vi "Draw.vi"(8 "error in (no error)":errorcluster, 11 "reference in":refnum<class "Pgui_Obj.lvclass">) -> (0 "error out":errorcluster, 2 "Draw Instr":picture, 3 "reference out":refnum<class "Pgui_Obj.lvclass">)   [LabVIEW 2019, in "Pgui_Obj.lvclass"]
uses:
  Pgui_Obj.lvclass
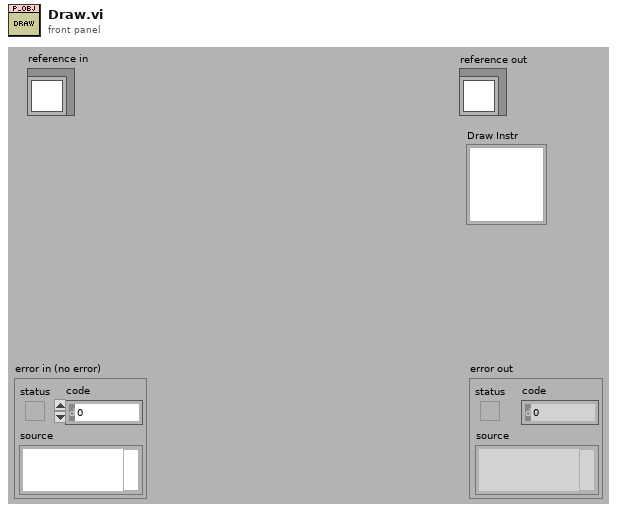
[diagram p1: front panel]
types:
  T1 = typedef "Pgui_Obj.lvclass/ObjectAttributes.ctl" = cluster{"Children":refnum<class "Pgui_Obj.lvclass">[], "Draw Instr":picture, "Params":cluster{"left":i16, "top":i16, "right":i16, "bottom":i16}, "Parent_Pgui_Obj":refnum<class "Pgui_Obj.lvclass">, "MouseOver":bool}
  T2 = cluster{"left":i16, "top":i16, "right":i16, "bottom":i16}
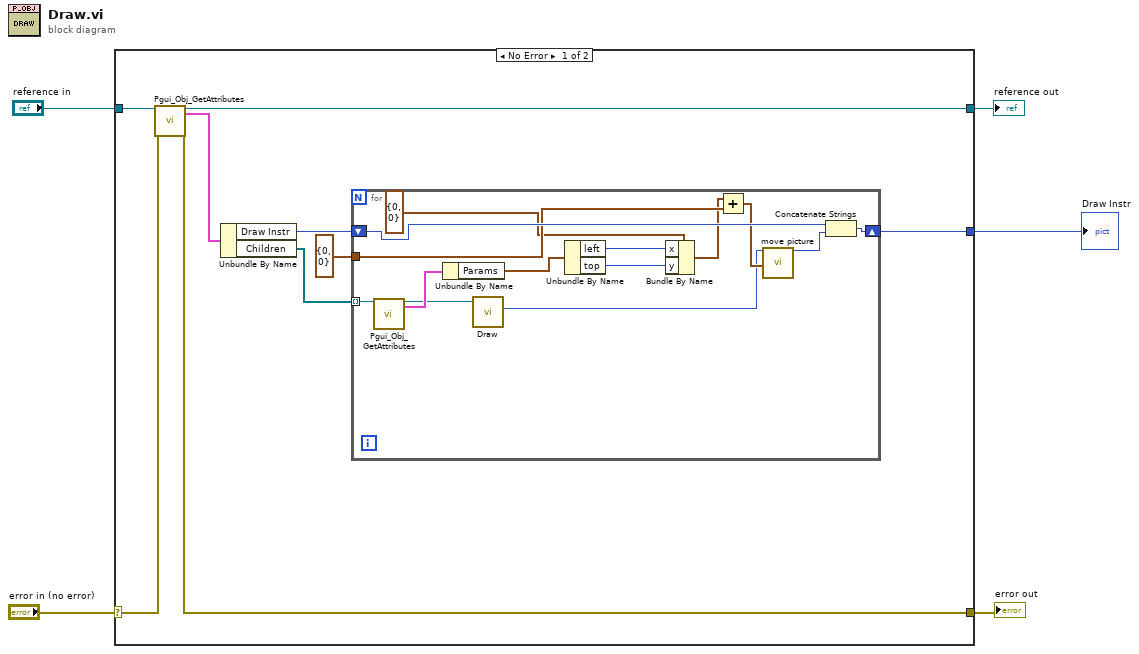
[diagram p0: block diagram]
diagram:
  n1 = case shown="No Error" "error in (no error)" {
    selector: "error in (no error)" -> [w14 w30]
    tunnel: [w12 w30] -> w4
    tunnel: [w10 w29] -> w2
    tunnel: "reference in" -> [w11 w29]
    tunnel: [w6 _] -> w1
    frame No Error {
      n2 = call "Pgui_Obj_GetAttributes.vi"("reference in"=w11, "error in (no error)"=w14) -> ("reference out"=w10:refnum<class "Pgui_Obj.lvclass">, "Data"=w13:T1, "error out"=w12:errorcluster)  [unwired: 14 in, 1 out]
      n3 = Unbundle By Name(w13) -> ("Draw Instr"=w9:picture, "Children"=w7:refnum<class "Pgui_Obj.lvclass">[])
      n4 = for {
        tunnel: w7 -> [w18] mode=indexing
        shift-right: [w28] -> w6
        shift-left: w9 -> [w26]
        tunnel: cluster{"x":i16, "y":i16} {"x"=0, "y"=0} ("input cluster") -> [w22]
        n5 = call "Pgui_Obj_GetAttributes.vi"("reference in"=w18) -> ("reference out"=w16:refnum<class "Pgui_Obj.lvclass">, "Data"=w17:T1)  [unwired: 15 in, 2 out]
        n6 = Unbundle By Name(w17) -> ("Params"=w25:T2)
        n7 = call-dynamic "Draw.vi"("reference in"=w16) -> ("Draw Instr"=w15:picture)  [unwired: 8 in, 2 out]
        n8 = Unbundle By Name(w25) -> ("left"=w24:i16, "top"=w23:i16)
        n9 = Bundle By Name(cluster=cluster{"x":i16, "y":i16} {"x"=0, "y"=0} ("move"), "x"=w24, "y"=w23) -> (w21:cluster{"x":i16, "y":i16})
        n10 = Add(x=w21, y=w22) -> (x+y=w19:cluster{"x":i16, "y":i16})
        n11 = call "move picture.vi"("Picture in"=w15, "move"=w19) -> ("Picture out"=w27:picture)  [unwired: 17 in]
        n12 = Concatenate Strings(w26, w27) -> (w28:picture)
      }
    }
    frame Error {
    }
  }
  "error out" <- w4
  "reference out" <- w2
  "Draw Instr" <- w1
